vi "Home Reference.vi"(8 "Error in":errorcluster, 11 "INL DNL Test in":refnum<class "INL DNL Test.lvclass">) -> (0 "Error out":errorcluster, 2 "VI Ref":refnum<vi>, 3 "INL DNL Test out":refnum<class "INL DNL Test.lvclass">)   [LabVIEW 2020, in "INL DNL Test.lvclass"]
doc: "Runs the home page asynchronously."
uses:
  INL DNL Test.lvclass
  Parent/Typedef/LV2 Control.ctl
  Home Page.vi
  Parent/Test.lvclass
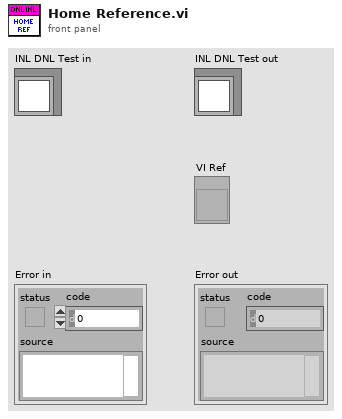
[diagram p1: front panel]
types:
  T1 = typedef "Test.lvclass/LV2 Control.ctl" = enum16{"Home", "Mode", "Config", "Status", "Read"}
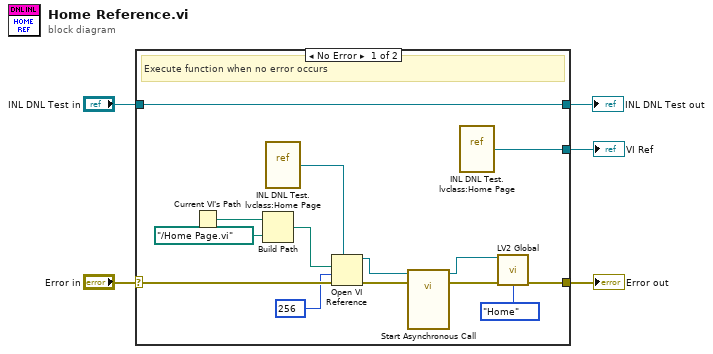
[diagram p0: block diagram]
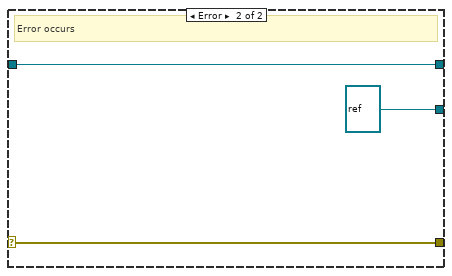
[diagram p2: hidden frame]
diagram:
  n1 = case shown="No Error" "Error in" {
    selector: "Error in" -> [w17 w22]
    tunnel: [w8 w22] -> w4
    tunnel: [w19 w21] -> w2
    tunnel: "INL DNL Test in" -> [w19 w21]
    tunnel: [w18 refnum<vi> refnum] -> w1
    frame No Error {
      # "Execute function when no error occurs"
      n2 = Current VI's Path() -> (path=w16:path)
      n3 = Build Path(base path=w16, name or relative path=path "../Home Page.vi") -> (appended path=w14:path)
      n4 = vi-ref "INL DNL Test.lvclass:Home Page.vi"() -> (w13:refnum<vi>)
      n5 = Open VI Reference(type specifier VI Refnum (for type only)=w13, vi path=w14, options=256, error in (no error)=w17) -> (vi reference=w12:refnum<vi>, error out=w11:errorcluster)  [unwired: 2 in]
      n6 = call-by-ref "Start Asynchronous Call"(reference=w12, error in=w11) -> (reference out=w6:refnum<vi>, error out=w9:errorcluster)  [unwired: 14 in, 2 out]
      n7 = vi-ref "INL DNL Test.lvclass:Home Page.vi"() -> (w18:refnum<vi>)
      n8 = call "LV2 Global.vi"("Home Ref In"=w6, "Error In"=w9, "Enum"=LV2_Control."Home") -> ("Error Out"=w8:errorcluster)  [unwired: 8 in, 4 out]
    }
    frame Error {
      # "Error occurs"
    }
  }
  "Error out" <- w4
  "INL DNL Test out" <- w2
  "VI Ref" <- w1
